vi "Uninitialize Attribute.vi"(8 "error in (no error)":errorcluster, 11 "Attribute.Config in":refnum<class "Attribute.Config.lvclass">) -> (0 "error out":errorcluster, 3 "Attribute.Config out":refnum<class "Attribute.Config.lvclass">)   [LabVIEW 2019, in "Attribute.Config.lvclass"]
doc: "JKI State Machine Objects (SMO) 1.3.0.56\nJKI - JKI\nCopyright (c) 2017, JKI"
uses:
  Attribute.Config.lvclass
  Attribute.Config.lvclass/Attribute.Config.ctl
  Attribute/Attribute.lvclass
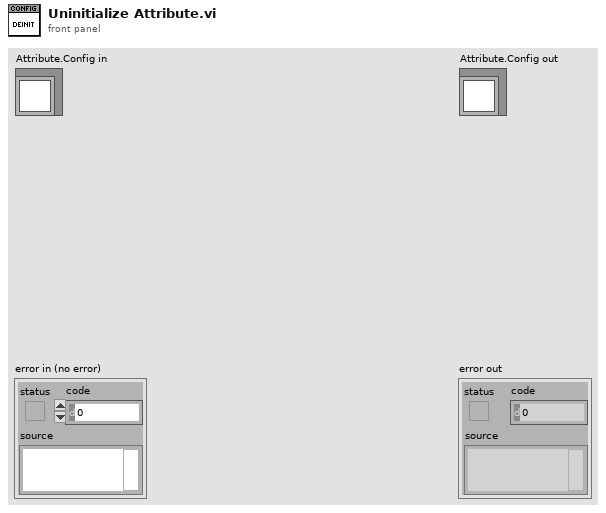
[diagram p1: front panel]
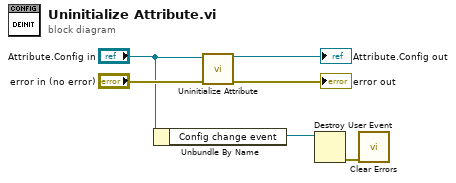
[diagram p0: block diagram]
diagram:
  n1 = Unbundle By Name("Attribute.Config in") -> ("Config change event"=w2:refnum<user-event>)
  n2 = call-parent "Uninitialize Attribute.vi"("error in (no error)"="error in (no error)", "Attribute in"="Attribute.Config in") -> ("error out"=→"error out":errorcluster, "Attribute out"=→"Attribute.Config out":refnum<class "Attribute.Config.lvclass">)  [unwired: 8 in]
  n3 = Destroy User Event(user event=w2) -> (error out=w1:errorcluster)  [unwired: 1 in]
  n4 = call <vilib>:"Clear Errors.vi"("error in (no error)"=w1) -> ()  [unwired: 5 in, 2 out]
